vi "WPI_DMAAddChannelToStream.vi"   [LabVIEW 2017]
doc: "Specifies the data transferred in the DMA stream. Wire a device reference from the other WPI Robotics Library Open VIs to specify the data you want to receive. The order that the AddChannel VIs add data to the DMA stream defines the order that the Read VI returns the data.\n\nYou must open a reference to a DMA stream with the Open VI before using this VI.\n\nThis software is licensed. Open the labview\\readme\\WPI Robotics Library Open Source License.txt file for more information."
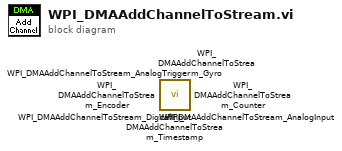
[diagram p0: block diagram]
diagram:
  n1 = call <vilib>:"WPI_DMAAddChannelToStream_Timestamp.vi"() -> ()  [unwired: 10 in, 2 out]
  n2 = call <vilib>:"WPI_DMAAddChannelToStream_Gyro.vi"() -> ()  [unwired: 10 in, 2 out]
  n3 = call <vilib>:"WPI_DMAAddChannelToStream_Encoder.vi"() -> ()  [unwired: 10 in, 2 out]
  n4 = call <vilib>:"WPI_DMAAddChannelToStream_Counter.vi"() -> ()  [unwired: 10 in, 2 out]
  n5 = call <vilib>:"WPI_DMAAddChannelToStream_AnalogTrigger.vi"() -> ()  [unwired: 10 in, 2 out]
  n6 = call <vilib>:"WPI_DMAAddChannelToStream_AnalogInput.vi"() -> ()  [unwired: 10 in, 2 out]
  n7 = call <vilib>:"WPI_DMAAddChannelToStream_DigitalInput.vi"() -> ()  [unwired: 10 in, 2 out]
